vi "Do.vi"(8 "error in (no error)":errorcluster, 10 "Actor in":refnum<class>, 11 "Message Template":refnum<class>) -> (0 "error out":errorcluster, 2 "Actor out":refnum<class>)   [LabVIEW 2023, in "Async Message Template Interface.lvclass"]
doc: "(<B>Filename</B>: Actor Framework.lvlib:Message.lvclass:Do.vi)\n\nDefines what a message does when it is received by an actor. Generally, a message instructs an actor to invoke one of its methods. By default, this method does nothing. A child class must override it to define behavior. Create a child class by using the Actor Framework Message Maker dialog box."
uses:
  Async Message Template Interface.lvclass
  Async Message Template Interface.lvclass/Async Message Template Interface.ctl
  8d21d422-f747-45dc-88b4-05fa8256bf27.vi
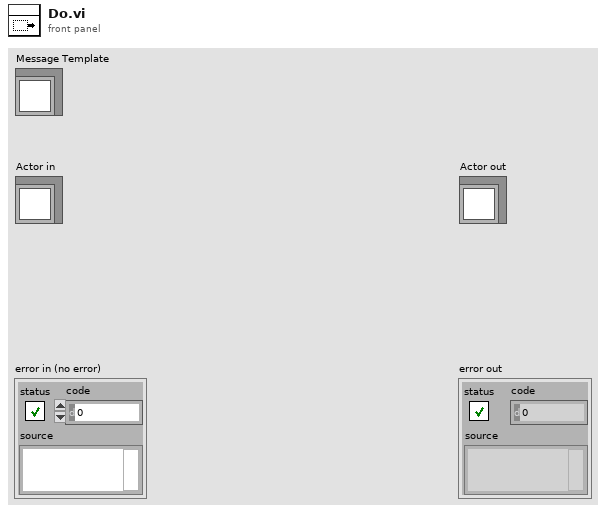
[diagram p1: front panel]
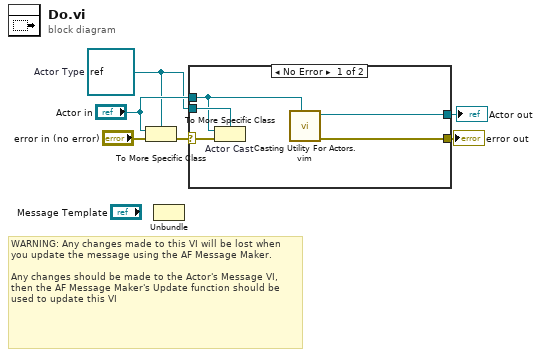
[diagram p0: block diagram]
diagram:
  w1 = refnum<class> refnum  # Actor Type
  # "WARNING: Any changes made to this VI will be lost when you update the message using the AF Message Maker.\n\nAny changes should be made to the Actor's Message VI, then the AF Message Maker's Update function should be used to update this VI"
  n1 = To More Specific Class(target class=w1, reference="Actor in", error in="error in (no error)") -> (error out=w5:errorcluster)  [unwired: 1 out]
  n2 = Unbundle() -> ()  [unwired: 1 in, 2 out]
  n3 = case shown="No Error" w5 {
    selector: w5 -> [w7 w13]
    tunnel: [w9 w13] -> w4
    tunnel: [w8 w12] -> w3
    tunnel: "Actor in" -> [w10 w12]
    tunnel: w1 -> [w11 _]
    frame No Error {
      n4 = To More Specific Class "Actor Cast"(target class=w11, reference=w10, error in=w7) -> ()  [unwired: 2 out]
      n5 = call "Casting Utility For Actors.vim"("type"=w10) -> ("error out"=w9:errorcluster, "Actor out"=w8:refnum<class>)  [unwired: 9 in]
    }
    frame Error {
    }
  }
  "error out" <- w4
  "Actor out" <- w3
